vi "Ramp down.vi"(8 "end power":dbl, 10 "Distance":dbl) -> (2 "power  out":dbl)   [LabVIEW 2017]
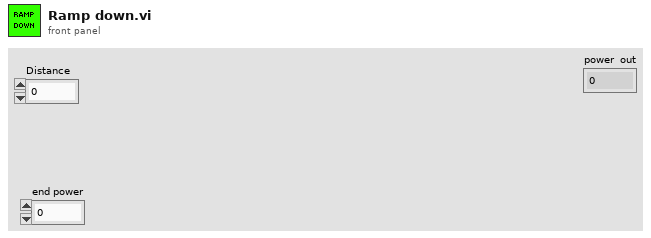
[diagram p1: front panel]
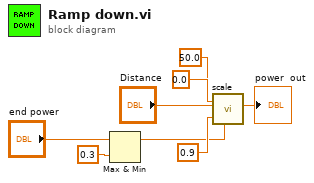
[diagram p0: block diagram]
diagram:
  n1 = Max & Min(x="end power", y=0.3) -> (max(x,y)=w1:dbl)  [unwired: 1 out]
  n2 = call "scale.vi"("Max"=0.9, "High"=50.0, "Min"=w1, "Low"=0.0, "In Signal"="Distance") -> ("Output signal"=→"power  out":dbl)  [unwired: 6 in]
